vi "Queue Registry.vi"(0 "method":T3, 5 "index (0)":i32, 9 "message queue in":T2, 11 "error in":errorcluster, 12 "properties in":T1) -> (3 "all properties":T1[](array[typedef]), 4 "all queues":T2[](array[typedef]), 6 "number of queues":i32, 10 "message queue out":T2, 14 "properties out":T1, 15 "error out":errorcluster)   [LabVIEW 2009, in "AMC.lvlib"]
doc: "Maintains the list of local message queues."
uses:
  AMC.lvlib
  Queue Registry Method.ctl
  Message Queue.ctl
  Message.ctl
  <vilib>/NI/Tools/Keyed Array/KeyedArray.ctl
  Queue Registry Properties.ctl
  <vilib>/NI/Tools/Keyed Array/Tools_KeyedArray.lvlib
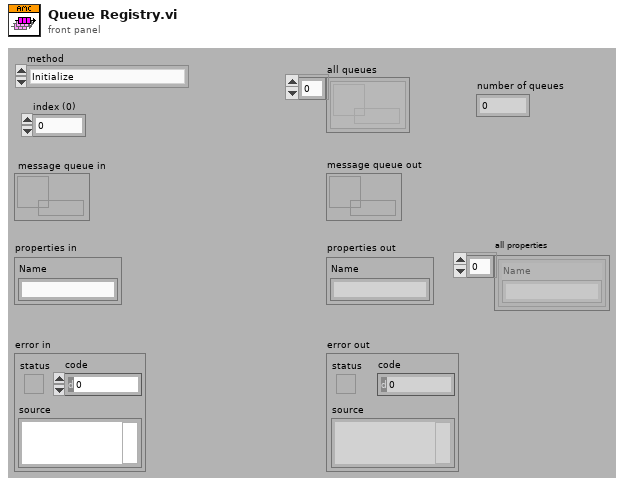
[diagram p1: front panel]
types:
  T1 = typedef "AMC.lvlib/Queue Registry Properties.ctl" = cluster{"Name":string}
  T2 = typedef "AMC.lvlib/Message Queue.ctl" = refnum<queue>
  T3 = typedef "AMC.lvlib/Queue Registry Method.ctl" = enum16{"Initialize", "Add Queue", "Set Properties", "Get Queue by Index", "Get Queue by Name", "Remove Queue", "Remove All Queues"}
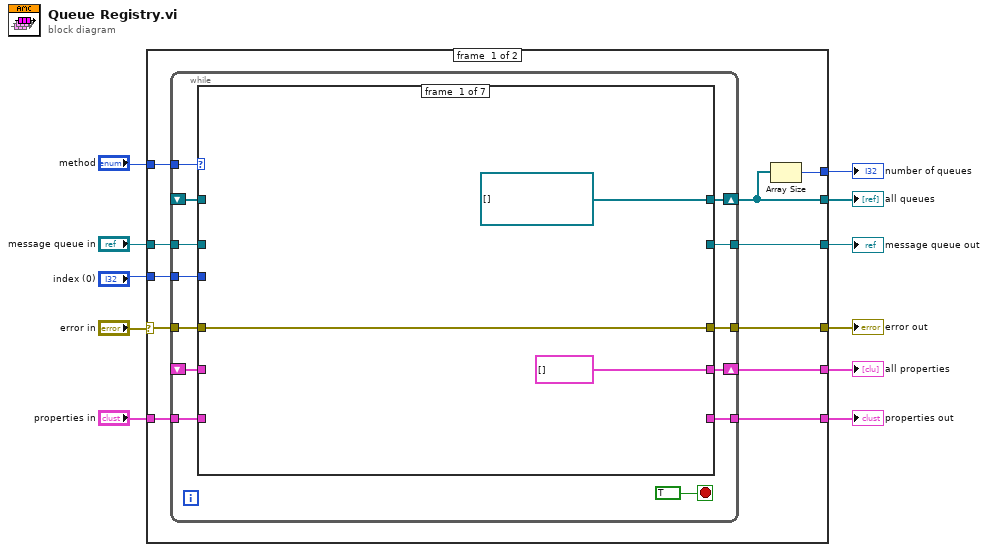
[diagram p0: block diagram]
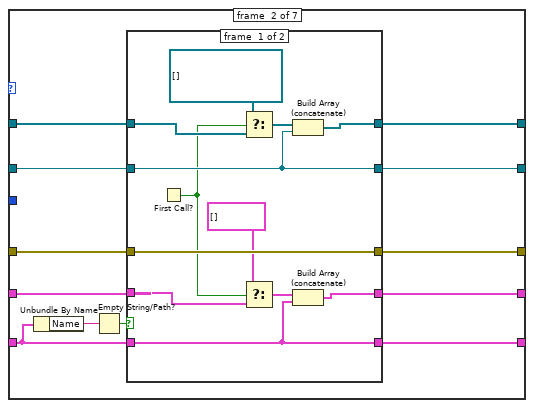
[diagram p2: hidden frame]
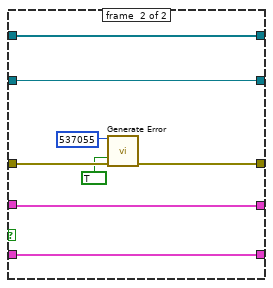
[diagram p3: hidden frame]
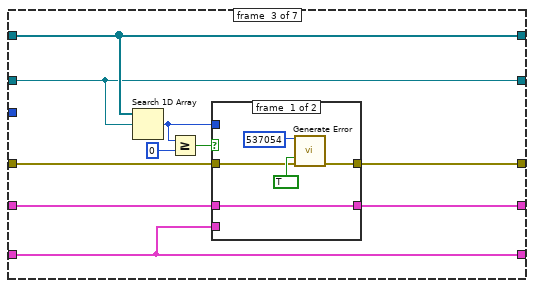
[diagram p4: hidden frame]
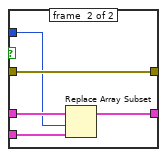
[diagram p5: hidden frame]
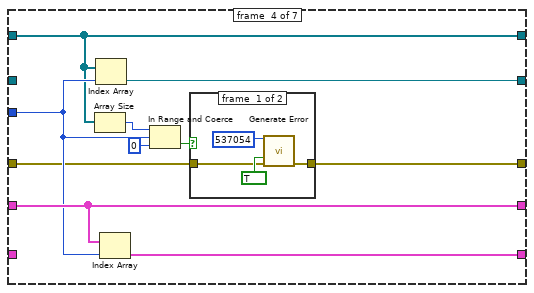
[diagram p6: hidden frame]
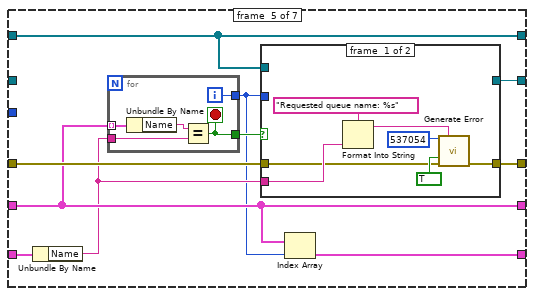
[diagram p8: hidden frame]
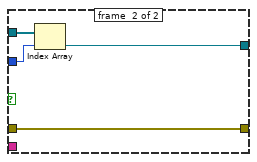
[diagram p9: hidden frame]
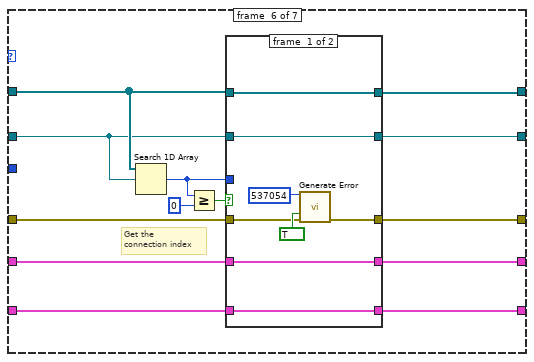
[diagram p10: hidden frame]
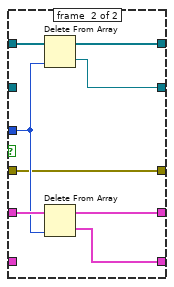
[diagram p11: hidden frame]
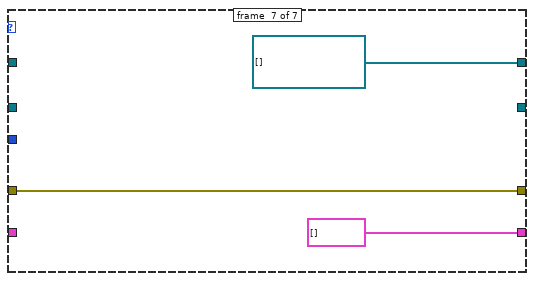
[diagram p12: hidden frame]
diagram:
  n1 = case shown="No Error" "error in" {
    selector: "error in" -> [w22 w165]
    tunnel: [w21 w165] -> w10
    tunnel: "index (0)" -> [w20 _]
    tunnel: "method" -> [w19 _]
    tunnel: "message queue in" -> [w18 w164]
    tunnel: [w12 _] -> w6
    tunnel: [w13 _] -> w5
    tunnel: [w17 w164] -> w4
    tunnel: "properties in" -> [w16 _]
    tunnel: [w15 _] -> w2
    tunnel: [w14 _] -> w1
    frame #0 {
      n2 = while {
        shift-right: [w28] -> w13
        shift-left: _ -> [w34]
        tunnel: w22 -> [w33]
        tunnel: [w32] -> w21
        tunnel: w20 -> [w31]
        tunnel: w19 -> [w30]
        tunnel: w18 -> [w29]
        tunnel: [w27] -> w17
        shift-right: [w24] -> w15
        shift-left: _ -> [w26]
        tunnel: w16 -> [w25]
        tunnel: [w23] -> w14
        stop <- TRUE stop-if-true
        n3 = case shown="\"Set Properties\"" w30 {
          tunnel: w34 -> [_ w47 w79 w96 w108 w144 _]
          tunnel: w29 -> [_ w49 w78 _ _ w136 _]
          tunnel: [T2[] [] w50 w79 w96 w108 w140 T2[] []] -> w28
          tunnel: [_ w43 w78 w100 w106 w139 _] -> w27
          tunnel: [w38 w41 w75 w91 w113 w138 w163] -> w32
          tunnel: w33 -> [w38 w40 w76 w94 w114 w137 w163]
          tunnel: w31 -> [_ _ _ w97 _ _ _]
          tunnel: w26 -> [_ w45 w74 w99 w110 w135 _]
          tunnel: w25 -> [_ w46 w71 _ w112 w132 _]
          tunnel: [T1[] [] w48 w72 w99 w110 w134 T1[] []] -> w24
          tunnel: [_ w42 w71 w98 w115 w133 _] -> w23
          frame #0 {
          }
          frame #1 {
            n4 = Unbundle By Name(w46) -> ("Name"=w39:string)
            n5 = Empty String/Path?(string/path=w39) -> (empty?=w44:bool)
            n6 = case shown="False" w44 {
              tunnel: [w62 w70] -> w50
              tunnel: w49 -> [w58 w69]
              tunnel: [w61 w68] -> w48
              tunnel: w47 -> [w60 w70]
              tunnel: w46 -> [w56 w67]
              tunnel: w45 -> [w59 w68]
              tunnel: [w58 w69] -> w43
              tunnel: [w56 w67] -> w42
              tunnel: [w57 w65] -> w41
              tunnel: w40 -> [w57 w66]
              frame #0 {
                n7 = First Call?() -> (First Call?: T/F=w52:bool)
                n8 = Select(t=T2[] [], s=w52, f=w60) -> (s? t:f=w55:T2[])
                n9 = Select(t=T1[] [], s=w52, f=w59) -> (s? t:f=w53:T1[])
                n10 = Build Array (concatenate)(w55, w58) -> (w62:T2[])
                n11 = Build Array (concatenate)(w53, w56) -> (w61:T1[])
              }
              frame #1 {
                n12 = call "Generate Error.vi"("code"=537055, "status (F)"=TRUE, "error in"=w66) -> ("error out"=w65:errorcluster)  [unwired: 12 in]
              }
            }
          }
          frame #2 {
            n13 = Search 1D Array(1D array=w79, element=w78) -> (index of element=w73:i32)  [unwired: 1 out]
            n14 = Greater Or Equal?(x=w73, y=0) -> (x >= y?=w77:bool)
            n15 = case shown="True" w77 {
              tunnel: w76 -> [w82 w90]
              tunnel: [w81 w90] -> w75
              tunnel: w74 -> [w85 w89]
              tunnel: w73 -> [_ w88]
              tunnel: w71 -> [_ w87]
              tunnel: [w85 w86] -> w72
              frame #0 {
                n16 = call "Generate Error.vi"("code"=537054, "status (F)"=TRUE, "error in"=w82) -> ("error out"=w81:errorcluster)  [unwired: 12 in]
              }
              frame #1 {
                n17 = Replace Array Subset(array=w89, new element=w87, index=w88) -> (w86:T1[])
              }
            }
          }
          frame #3 {
            n18 = Array Size(array=w96) -> (size(s)=w95:i32)
            n19 = Index Array(array=w96, index=w97) -> (element=w100:T2)
            n20 = Index Array(array=w99, index=w97) -> (element=w98:T1)
            n21 = In Range and Coerce(upper limit=w95, x=w97, lower limit=0) -> (In Range?=w93:bool)  [unwired: 1 out]
            n22 = case shown="False" w93 {
              tunnel: w94 -> [w102 w105]
              tunnel: [w101 w105] -> w91
              frame #0 {
                n23 = call "Generate Error.vi"("code"=537054, "status (F)"=TRUE, "error in"=w102) -> ("error out"=w101:errorcluster)  [unwired: 12 in]
              }
              frame #1 {
              }
            }
          }
          frame #4 {
            n24 = Unbundle By Name(w112) -> ("Name"=w109:string)
            n25 = for {
              tunnel: w110 -> [w120] mode=indexing
              tunnel: w109 -> [w118]
              tunnel: [w117] -> w111
              tunnel: [w116] -> w107
              i -> [w116]
              stop <- w117 stop-if-true
              n26 = Unbundle By Name(w120) -> ("Name"=w119:string)
              n27 = Equal?(x=w119, y=w118) -> (x = y?=w117:bool)
            }
            n28 = case shown="False" w111 {
              tunnel: w114 -> [w123 w131]
              tunnel: [w121 w131] -> w113
              tunnel: w109 -> [w126 _]
              tunnel: w108 -> [_ w130]
              tunnel: w107 -> [_ w129]
              tunnel: [_ w128] -> w106
              frame #0 {
                n29 = Format Into String(format string="Requested queue name: %s" ("source"), w126) -> (resulting string=w122:string)  [unwired: 2 in, 1 out]
                n30 = call "Generate Error.vi"("code"=537054, "<append> (\"\")"=w122, "status (F)"=TRUE, "error in"=w123) -> ("error out"=w121:errorcluster)  [unwired: 11 in]
              }
              frame #1 {
                n31 = Index Array(array=w130, index=w129) -> (element=w128:T2)
              }
            }
            n32 = Index Array(array=w110, index=w107) -> (element=w115:T1)
          }
          frame #5 {
            # "Get the \nconnection index"
            n33 = Search 1D Array(1D array=w144, element=w136) -> (index of element=w143:i32)  [unwired: 1 out]
            n34 = Greater Or Equal?(x=w143, y=0) -> (x >= y?=w141:bool)
            n35 = case shown="True" w141 {
              tunnel: w144 -> [w152 w159]
              tunnel: w143 -> [_ w156]
              tunnel: [w152 w160] -> w140
              tunnel: [w151 w154] -> w139
              tunnel: [w145 w153] -> w138
              tunnel: w137 -> [w146 w153]
              tunnel: w136 -> [w151 _]
              tunnel: w135 -> [w150 w158]
              tunnel: [w150 w157] -> w134
              tunnel: [w149 w155] -> w133
              tunnel: w132 -> [w149 _]
              frame #0 {
                n36 = call "Generate Error.vi"("code"=537054, "status (F)"=TRUE, "error in"=w146) -> ("error out"=w145:errorcluster)  [unwired: 12 in]
              }
              frame #1 {
                n37 = Delete From Array(array=w159, index=w156) -> (deleted portion=w154:T2, array with subset deleted=w160:T2[])  [unwired: 1 in]
                n38 = Delete From Array(array=w158, index=w156) -> (deleted portion=w155:T1, array with subset deleted=w157:T1[])  [unwired: 1 in]
              }
            }
          }
          frame #6 {
          }
        }
      }
      n39 = Array Size(array=w13) -> (size(s)=w12:i32)
    }
    frame #1 {
    }
  }
  "error out" <- w10
  "number of queues" <- w6
  "all queues" <- w5
  "message queue out" <- w4
  "all properties" <- w2
  "properties out" <- w1
